vi "Onset (SubVI).vi"(1 "bool_in_prev":bool, 2 "bool_in":bool) -> (0 "Onset":bool)   [LabVIEW 2013]
doc: "Based on the current and previous value of a boolean value, determine if it has just changed to true (\"onset\") or not.\n\nTruth table:\nPrevious value | Current value | Onset\nTrue | True | False\nTrue | False | False\nFalse | True | True\nFalse | False | False"
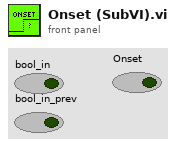
[diagram p1: front panel]
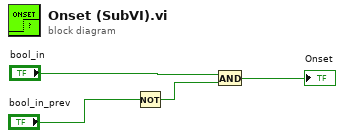
[diagram p0: block diagram]
diagram:
  n1 = Not(x="bool_in_prev") -> (.not. x?=w2:bool)
  n2 = And(x="bool_in", y=w2) -> (x .and. y?=→"Onset":bool)
